vi "File Viewer v3.vi"() -> ()   [LabVIEW 2019]
uses:
  <vilib>/Utility/file.llb/Read Delimited Spreadsheet (I64).vi
panel:
  in  "Stop":bool
  in  "Tab Control":T1(tab)
  out "Raw Image From Camera":i32[][](graph)
  in  "file path for picture":path
  out "Expected position on spectrometer (pixels):":dbl
  in  "Grating:":u16(ring) items=["Shimadzu 30-006  "]
  in  "Laser:":u16(ring) items=["800nm  "]
  in  "Harmonic":dbl min=10.0 max=40.0
  out "l (nm)":dbl
  out "E (J)":dbl
  out "E (eV)":dbl
  out "Nearest Harmonic of 800nm":dbl
  out "Vertical Binned Waveform Graph":i64[](graph)
  out "Cursor Position (pixels)":dbl
  out "Distance to nearest harmonic of 800nm (pixels)":dbl
  in  "Caibration Date":u16(ring) items=["first calibration - 7/31", "7/31-current"]
  out "Wavelength Graph":cluster{"lamda (m)":dbl, "Numeric":i64}[](graph)
  out "Energy Graph (eV)":cluster{"lamda (m)":dbl, "Numeric":i64}[](graph)
  out "Harmonics Graph":cluster{"lamda (m)":dbl, "Numeric":i64}[](graph)
  in  "Pump/Probe Run Folder:":path
  out "Distance to nearest harmonic of 800nm (pixels)":dbl
  out "Cursor Position on CCD  (pixels)":dbl
  out "Nearest Harmonic of 800nm":dbl
  out "E (eV) 2":dbl
  out "E (J)":dbl
  out "l (nm)":dbl
  in  "Pump/Probe Harmonic:":dbl min=10.0 max=40.0
  out "Expected position on spectrometer (pixels):":dbl
  out "Time delay":dbl
  out "XUV":dbl[][](graph)
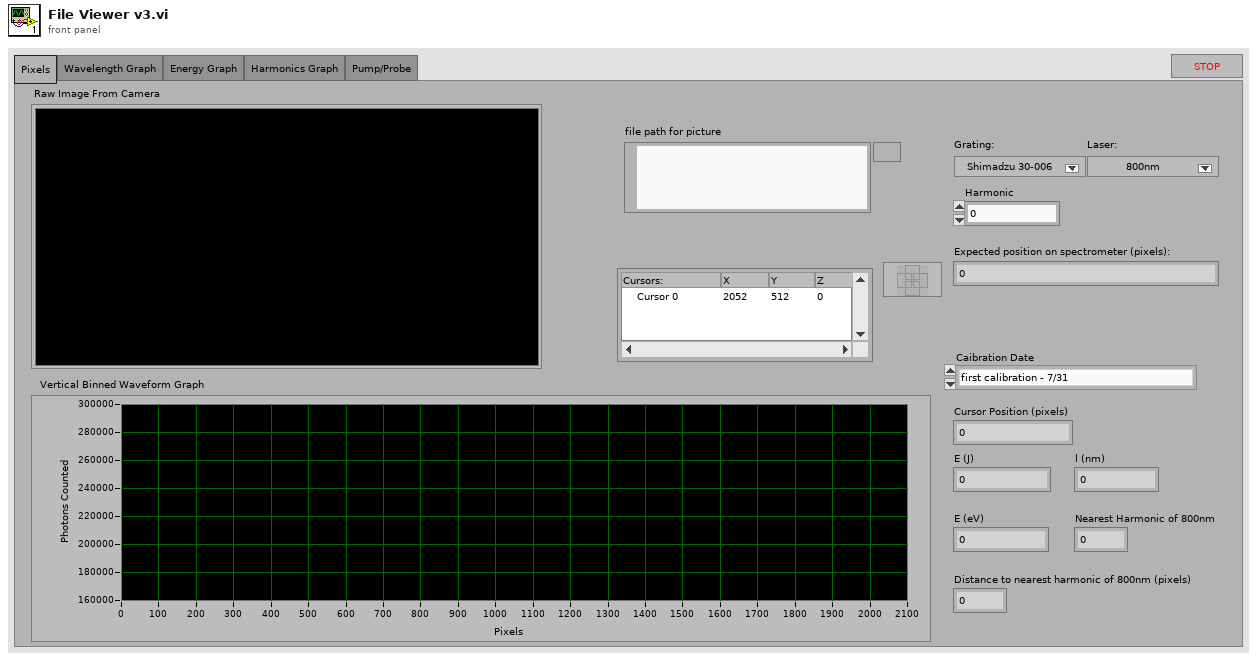
[diagram p1: front panel]
types:
  T1 = enum32{"Pixels", "Wavelength Graph", "Energy Graph", "Harmonics Graph", "Pump/Probe"}
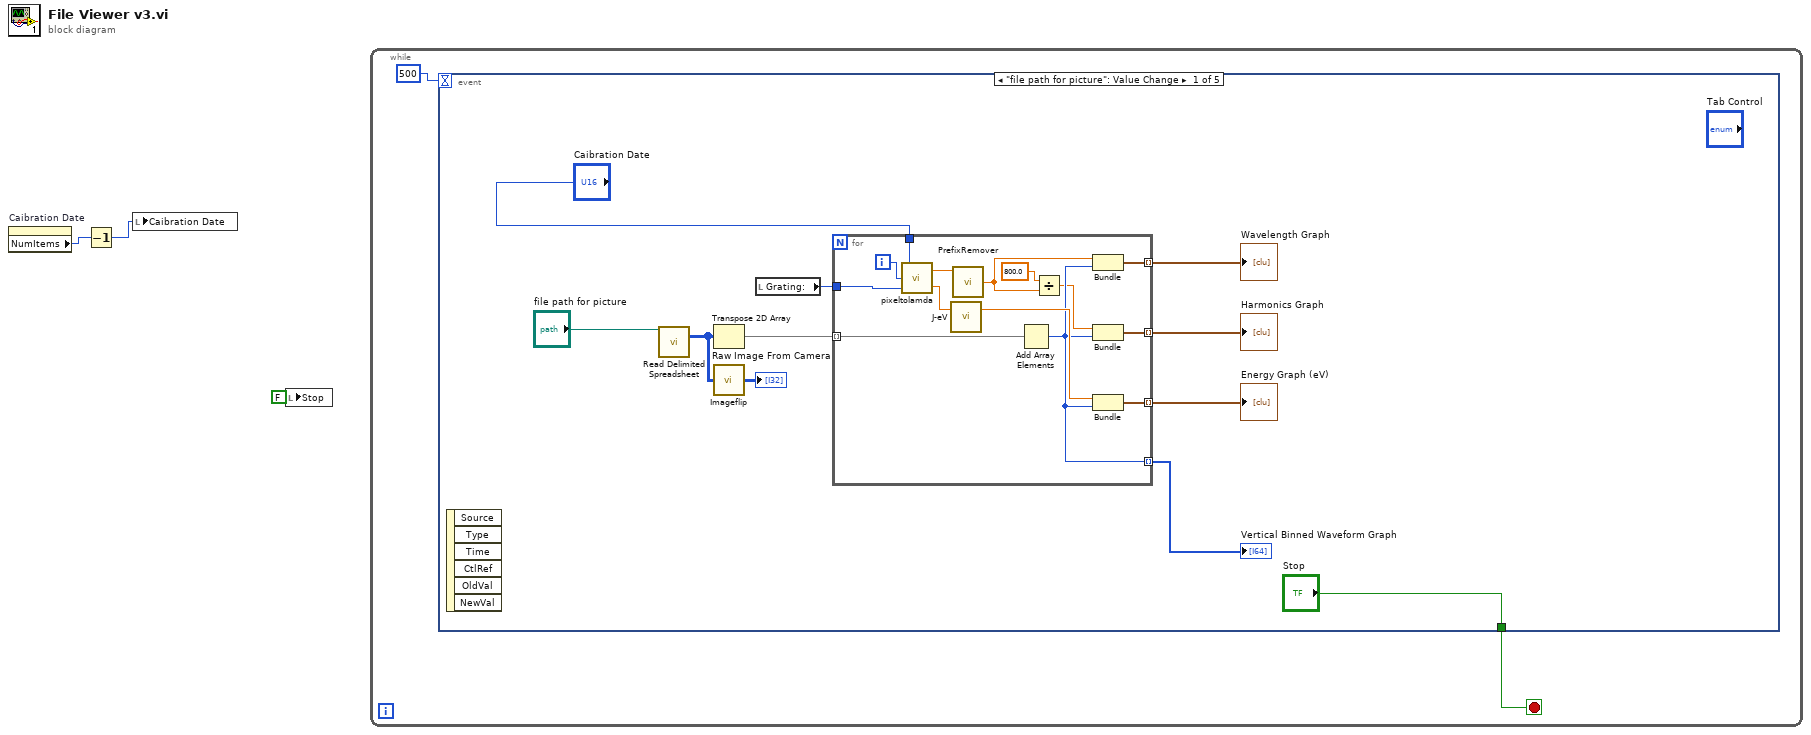
[diagram p0: block diagram]
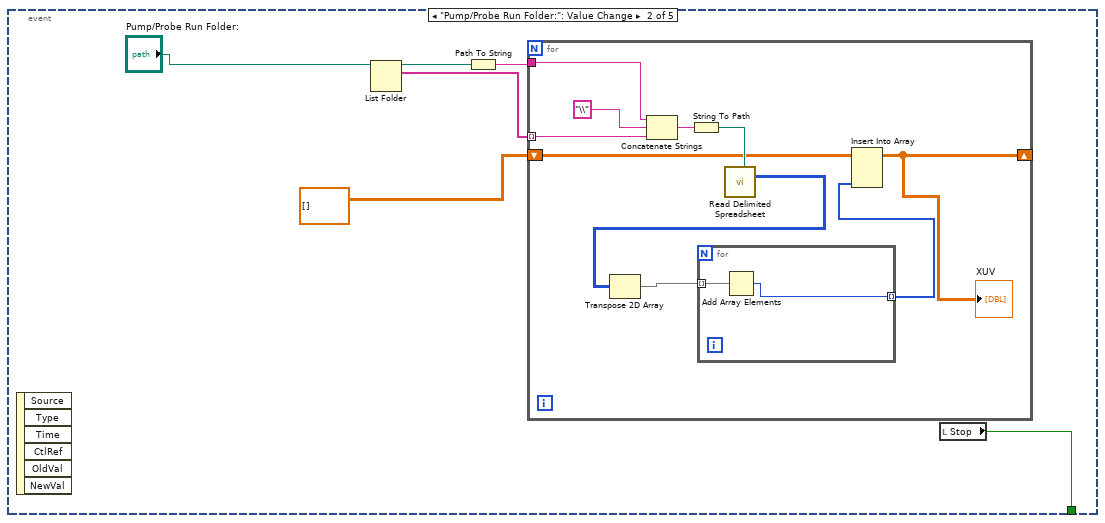
[diagram p2: hidden frame]
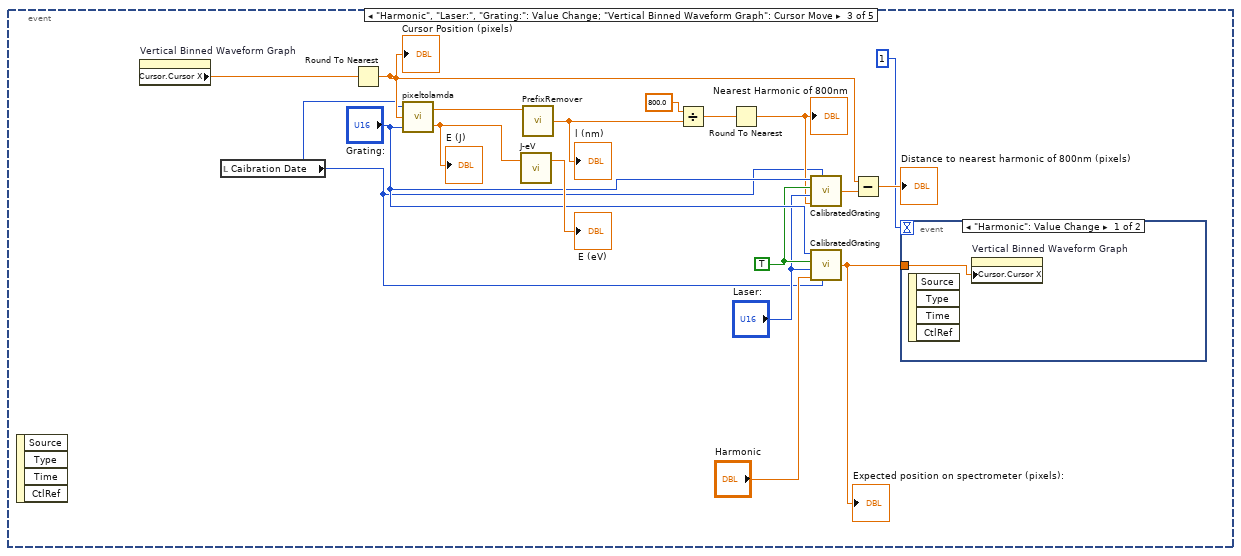
[diagram p3: hidden frame]
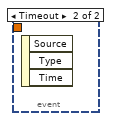
[diagram p4: hidden frame]
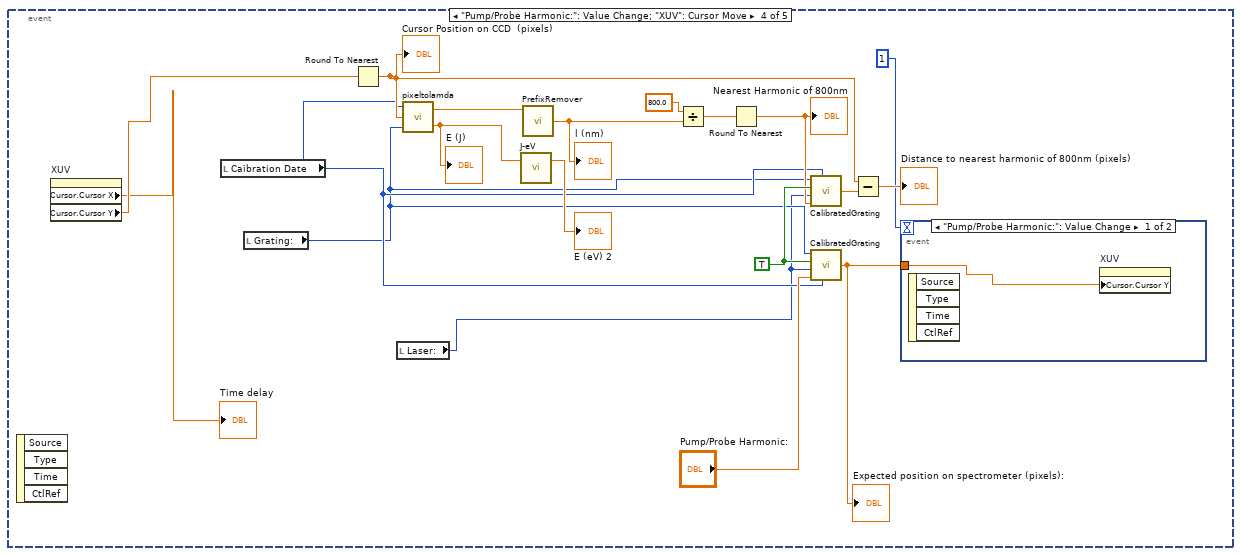
[diagram p5: hidden frame]
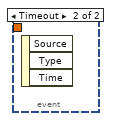
[diagram p6: hidden frame]
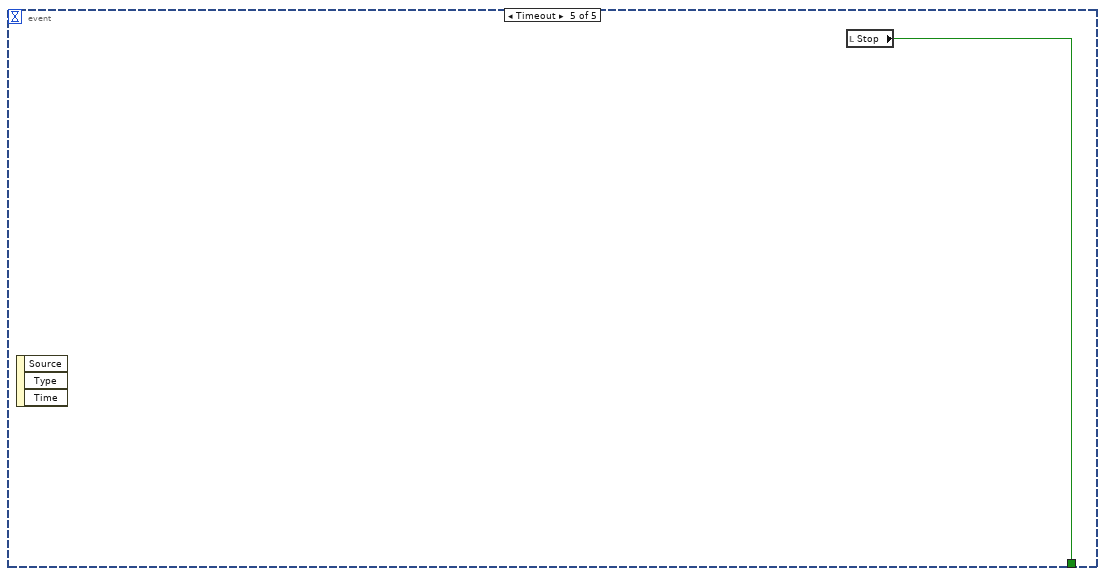
[diagram p7: hidden frame]
diagram:
  n1 = property on="Caibration Date" class="Ring (strict)"() -> ("NumItems"=w1:u32)  [unwired: 2 in, 2 out]
  n2 = Decrement(x=w1) -> (x-1=w2:u32)
  n3 = local write "Caibration Date"(w2) -> ()
  n4 = local write "Stop"(FALSE) -> ()
  n5 = while {
    stop <- w5 stop-if-true
    n6 = event shown="[0] \"file path for picture\": Value Change" {
      selector: _ -> [_ _ _ _ _]
      dyn-events: _ -> [_ _ _ _ _]
      timeout: 500 -> [_ _ _ _ _]
      tunnel: ["Stop" w32 _ _ w88] -> w5
      event "file path for picture": Value Change {
        n7 = event-data() -> ()  [unwired: 1 in, 6 out]
        n8 = call-poly <vilib>:"Read Delimited Spreadsheet.vi"("file path (dialog if empty)"="file path for picture") -> ("all rows"=w13:i64[][])  [unwired: 9 in, 5 out]
        n9 = Transpose 2D Array(2D array=w13) -> (transposed array=w12:i64[][])
        n10 = call "Imageflip.vi"("2D array"=w13) -> ("transposed array"=→"Raw Image From Camera":i32[][])
        n11 = local read "Grating:"() -> (w10:u16)
        n12 = for {
          tunnel: w12 -> [w30] mode=indexing
          tunnel: [w23] -> w11 mode=indexing
          tunnel: w10 -> [w28]
          tunnel: [w27] -> w9 mode=indexing
          tunnel: [w24] -> w8 mode=indexing
          tunnel: [w18] -> w7 mode=indexing
          tunnel: "Caibration Date" -> [w17]
          i -> [w29]
          n13 = call "pixeltolamda.vi"("Grating:"=w28, "Pixel Postion"=w29, "Caibration Date"=w17) -> ("E (J)"=w26:dbl, "lamda (m)"=w21:dbl)
          n14 = call "J-eV.vi"("J"=w26) -> ("eV"=w25:dbl)  [unwired: 1 in, 1 out]
          n15 = call "PrefixRemover.vi"("Nano"=w21) -> ("No prefix"=w20:dbl)  [unwired: 3 in]
          n16 = Add Array Elements(numeric array=w30) -> (sum=w23:i64)
          n17 = Divide(x=800.0, y=w20) -> (x/y=w19:dbl)
          n18 = Bundle("No prefix"=w20, "Numeric"=w23) -> (w27:cluster{"No prefix":dbl, "Numeric":i64})  [unwired: 1 in]
          n19 = Bundle(w19, "Numeric"=w23) -> (w18:cluster{dbl, "Numeric":i64})  [unwired: 1 in]
          n20 = Bundle("eV"=w25, "Numeric"=w23) -> (w24:cluster{"eV":dbl, "Numeric":i64})  [unwired: 1 in]
        }
        "Vertical Binned Waveform Graph" <- w11
        "Wavelength Graph" <- w9
        "Energy Graph (eV)" <- w8
        "Harmonics Graph" <- w7
      }
      event "Pump/Probe Run Folder:": Value Change {
        n21 = event-data() -> ()  [unwired: 1 in, 6 out]
        n22 = List Folder(path="Pump/Probe Run Folder:") -> (path out=w34:path, filenames=w35:string[])  [unwired: 3 in, 2 out]
        n23 = Path To String(path=w34) -> (string=w33:string)
        n24 = for {
          tunnel: w35 -> [w44] mode=indexing
          tunnel: w33 -> [w42]
          shift-right: [w37] -> _
          shift-left: dbl[][] [] -> [w41]
          n25 = Concatenate Strings(w42, "\\" ("string"), w44) -> (w46:string)
          n26 = String To Path(string=w46) -> (path=w45:path)
          n27 = call-poly <vilib>:"Read Delimited Spreadsheet.vi"("file path (dialog if empty)"=w45) -> ("all rows"=w39:i64[][])  [unwired: 9 in, 5 out]
          n28 = Transpose 2D Array(2D array=w39) -> (transposed array=w38:i64[][])
          n29 = for {
            tunnel: w38 -> [w48] mode=indexing
            tunnel: [w47] -> w40 mode=indexing
            n30 = Add Array Elements(numeric array=w48) -> (sum=w47:i64)
          }
          n31 = Insert Into Array(array=w41, new element=w40) -> (w37:dbl[][])  [unwired: 2 in]
          "XUV" <- w37
        }
        n32 = local read "Stop"() -> (w32:bool)
      }
      event "Harmonic", "Laser:", "Grating:": Value Change; "Vertical Binned Waveform Graph": Cursor Move {
        w58 = TRUE ("Subvi?")
        n33 = event-data() -> ()  [unwired: 1 in, 4 out]
        n34 = property on="Vertical Binned Waveform Graph" class="WFGraph (strict)"() -> ("Cursor.Cursor X"=w60:dbl)  [unwired: 2 in, 2 out]
        n35 = local read "Caibration Date"() -> (w49:u16)
        n36 = Round To Nearest(number=w60) -> (nearest integer value=w52:dbl)
        "Cursor Position (pixels)" <- w52
        n37 = call "pixeltolamda.vi"("Grating:"="Grating:", "Pixel Postion"=w52, "Caibration Date"=w49) -> ("E (J)"=w64:dbl, "lamda (m)"=w65:dbl)
        "E (J)" <- w64
        n38 = call "J-eV.vi"("J"=w64) -> ("eV"=→"E (eV)":dbl)  [unwired: 1 in, 1 out]
        n39 = call "PrefixRemover.vi"("Nano"=w65) -> ("No prefix"=w55:dbl)  [unwired: 3 in]
        "l (nm)" <- w55
        n40 = Divide(x=800.0, y=w55) -> (x/y=w62:dbl)
        n41 = Round To Nearest(number=w62) -> (nearest integer value=w56:dbl)
        "Nearest Harmonic of 800nm" <- w56
        n42 = call "CalibratedGrating.vi"("Grating:"="Grating:", "Subvi?"=w58, "Laser:"="Laser:", "Harmonic"=w56, "Caibration Date"=w49) -> ("Position on spectrometer (pixels):"=w54:dbl)
        n43 = call "CalibratedGrating.vi"("Grating:"="Grating:", "Subvi?"=w58, "Laser:"="Laser:", "Harmonic"="Harmonic", "Caibration Date"=w49) -> ("Position on spectrometer (pixels):"=w51:dbl)
        "Expected position on spectrometer (pixels):" <- w51
        n44 = Subtract(x=w52, y=w54) -> (x-y=→"Distance to nearest harmonic of 800nm (pixels)":dbl)
        n45 = event shown="[0] \"Harmonic\": Value Change" {
          selector: _ -> [_ _]
          dyn-events: _ -> [_ _]
          timeout: 1 -> [_ _]
          tunnel: w51 -> [w67 _]
          event "Harmonic": Value Change {
            n46 = event-data() -> ()  [unwired: 1 in, 4 out]
            n47 = property on="Vertical Binned Waveform Graph" class="WFGraph (strict)"("Cursor.Cursor X"=w67) -> ()  [unwired: 2 in, 2 out]
          }
          event Timeout {
            n48 = event-data() -> ()  [unwired: 1 in, 3 out]
          }
        }
      }
      event "Pump/Probe Harmonic:": Value Change; "XUV": Cursor Move {
        w80 = TRUE ("Subvi?")
        n49 = event-data() -> ()  [unwired: 1 in, 4 out]
        n50 = property on="XUV" class="IntGraph (strict)"() -> ("Cursor.Cursor X"=→"Time delay":dbl, "Cursor.Cursor Y"=w69:dbl)  [unwired: 2 in, 2 out]
        n51 = local read "Caibration Date"() -> (w72:u16)
        n52 = local read "Grating:"() -> (w71:u16)
        n53 = Round To Nearest(number=w69) -> (nearest integer value=w75:dbl)
        "Cursor Position on CCD  (pixels)" <- w75
        n54 = local read "Laser:"() -> (w70:u16)
        n55 = call "pixeltolamda.vi"("Grating:"=w71, "Pixel Postion"=w75, "Caibration Date"=w72) -> ("E (J)"=w84:dbl, "lamda (m)"=w85:dbl)
        "E (J)" <- w84
        n56 = call "J-eV.vi"("J"=w84) -> ("eV"=→"E (eV) 2":dbl)  [unwired: 1 in, 1 out]
        n57 = call "PrefixRemover.vi"("Nano"=w85) -> ("No prefix"=w78:dbl)  [unwired: 3 in]
        "l (nm)" <- w78
        n58 = Divide(x=800.0, y=w78) -> (x/y=w82:dbl)
        n59 = Round To Nearest(number=w82) -> (nearest integer value=w79:dbl)
        "Nearest Harmonic of 800nm" <- w79
        n60 = call "CalibratedGrating.vi"("Grating:"=w71, "Subvi?"=w80, "Laser:"=w70, "Harmonic"=w79, "Caibration Date"=w72) -> ("Position on spectrometer (pixels):"=w77:dbl)
        n61 = call "CalibratedGrating.vi"("Grating:"=w71, "Subvi?"=w80, "Laser:"=w70, "Harmonic"="Pump/Probe Harmonic:", "Caibration Date"=w72) -> ("Position on spectrometer (pixels):"=w74:dbl)
        "Expected position on spectrometer (pixels):" <- w74
        n62 = Subtract(x=w75, y=w77) -> (x-y=→"Distance to nearest harmonic of 800nm (pixels)":dbl)
        n63 = event shown="[0] \"Pump/Probe Harmonic:\": Value Change" {
          selector: _ -> [_ _]
          dyn-events: _ -> [_ _]
          timeout: 1 -> [_ _]
          tunnel: w74 -> [w87 _]
          event "Pump/Probe Harmonic:": Value Change {
            n64 = event-data() -> ()  [unwired: 1 in, 4 out]
            n65 = property on="XUV" class="IntGraph (strict)"("Cursor.Cursor Y"=w87) -> ()  [unwired: 2 in, 2 out]
          }
          event Timeout {
            n66 = event-data() -> ()  [unwired: 1 in, 3 out]
          }
        }
      }
      event Timeout {
        n67 = event-data() -> ()  [unwired: 1 in, 3 out]
        n68 = local read "Stop"() -> (w88:bool)
      }
    }
  }
